vi "Sender2.vi"() -> ()   [LabVIEW 2019]
uses:
  <vilib>/userDefined/High Color/IMAQdx.ctl
  <vilib>/vision/driver/NI_Vision_Acquisition_Software.lvlib
panel:
  in  "stop":bool
  out "Status":string
  out "Image":T1(plugin-control)
  in  "port":u16=3015
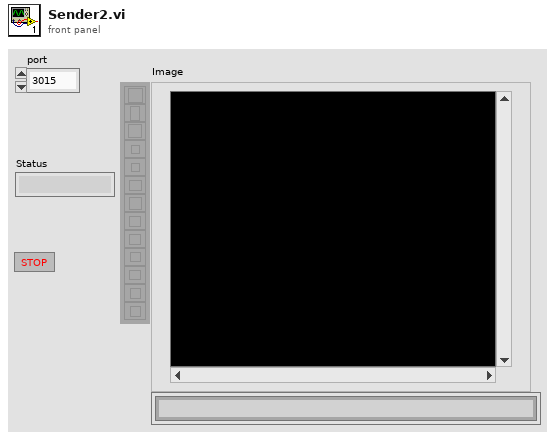
[diagram p1: front panel]
types:
  T1 = typedef "IMAQ Image.ctl" = refnum<image>
  T2 = typedef "IMAQdx.ctl" = refnum<k21>
  T3 = typedef "Image Type" = u32
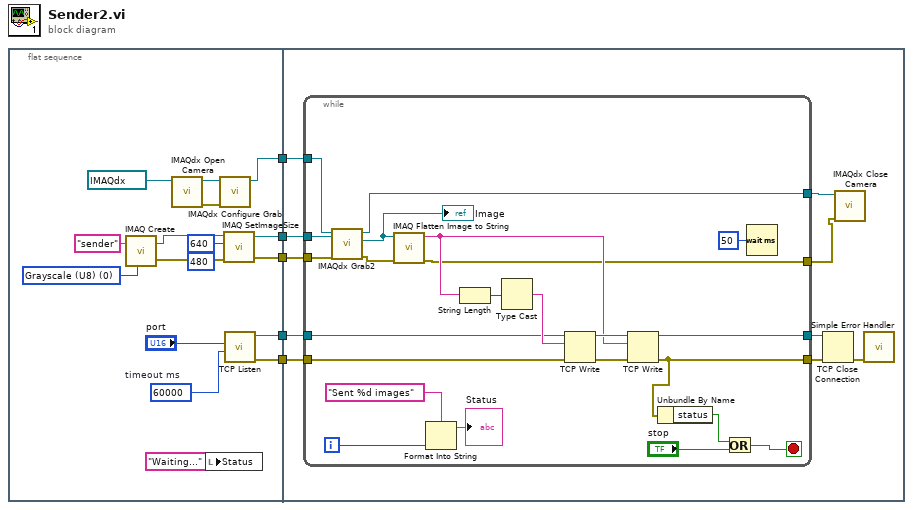
[diagram p0: block diagram]
diagram:
  n1 = flat-sequence {
    tunnel: [w14] -> w5
    tunnel: [w13] -> w4
    tunnel: [w16] -> w3
    tunnel: [w15] -> w2
    tunnel: [w6] -> w1
    tunnel: w5 -> [w32]
    tunnel: w4 -> [w31]
    tunnel: w3 -> [w30]
    tunnel: w2 -> [w29]
    tunnel: w1 -> [w25]
    frame #0 {
      w19 = 60000  # timeout ms
      w18 = T3 0 items=["Grayscale (U8)", "Grayscale (I16)", "Grayscale (SGL)", "Complex (CSG)", "RGB (U32)", "HSL (U32)", "RGB (U64)"] ("Image Type")
      n2 = call "IMAQ Create"("Image Name"="sender", "Image Type"=w18) -> ("New Image"=w21:T1, "error out"=w22:errorcluster)  [unwired: 3 in]
      n3 = call <vilib>:"IMAQdx Open Camera.vi"("Session In"=T2 "cam1") -> ("error out"=w7:errorcluster, "Session Out"=w8:T2)  [unwired: 9 in]
      n4 = local write "Status"("Waiting..." ("Status")) -> ()
      n5 = call <vilib>:"IMAQdx Configure Grab.vi"("error in"=w7, "Session In"=w8) -> ("Session Out"=w6:T2)  [unwired: 8 in, 1 out]
      n6 = call "IMAQ SetImageSize"("error in (no error)"=w22, "Y Resolution"=480, "X Resolution"=640, "Image"=w21) -> ("error out"=w15:errorcluster, "Image Out"=w16:T1)  [unwired: 1 in]
      n7 = call <vilib>:"TCP Listen.vi"("timeout ms (wait forever: -1)"=w19, "port"="port") -> ("error out"=w13:errorcluster, "connection ID"=w14:refnum<k5>)  [unwired: 5 in, 3 out]
    }
    frame #1 {
      n8 = while {
        tunnel: w32 -> [w53]
        tunnel: w31 -> [w52]
        tunnel: w30 -> [w38]
        tunnel: w29 -> [w36]
        tunnel: [w42] -> w28
        tunnel: [w41] -> w26
        tunnel: w25 -> [w39]
        tunnel: [w34] -> w24
        tunnel: [w33] -> w23
        i -> [w44]
        stop <- w47 stop-if-true
        n9 = call <vilib>:"IMAQdx Grab2.vi"("error in"=w36, "Image In"=w38, "Session In"=w39) -> ("error out"=w35:errorcluster, "Image Out"=w37:T1, "Session Out"=w34:T2)  [unwired: 5 in, 1 out]
        "Image" <- w37
        n10 = call "IMAQ Flatten Image to String"("error in (no error)"=w35, "Image"=w37) -> ("error out"=w33:errorcluster, "Data String"=w49:string)  [unwired: 8 in]
        n11 = Format Into String(format string="Sent %d images", w44) -> (resulting string=→"Status":string)  [unwired: 2 in, 1 out]
        n12 = String Length(string=w49) -> (length=w55:i32)
        n13 = Type Cast(x=w55) -> (*(type *) &x=w54:string)  [unwired: 1 in]
        n14 = TCP Write(connection ID=w53, data in=w54, error in (no error)=w52) -> (connection ID out=w51:refnum<k5>, error out=w50:errorcluster)  [unwired: 1 in, 1 out]
        n15 = TCP Write(connection ID=w51, data in=w49, error in (no error)=w50) -> (connection ID out=w41:refnum<k5>, error out=w42:errorcluster)  [unwired: 1 in, 1 out]
        n16 = Unbundle By Name(w42) -> ("status"=w46:bool)
        n17 = Or(x=w46, y="stop") -> (x .or. y?=w47:bool)
        n18 = Wait (ms)(milliseconds to wait=u32 50) -> ()  [unwired: 1 out]
      }
      n19 = TCP Close Connection(connection ID=w26, error in (no error)=w28) -> (error out=w27:errorcluster)  [unwired: 1 in, 1 out]
      n20 = call <vilib>:"IMAQdx Close Camera.vi"("error in"=w23, "Session In"=w24) -> ()  [unwired: 9 in, 1 out]
      n21 = call <vilib>:"Simple Error Handler.vi"("error in (no error)"=w27) -> ()  [unwired: 4 in, 5 out]
    }
  }
